vi "SetTriggerDelay.vi"(8 "error in (no error)":errorcluster, 10 "Arg":string, 11 "ThorLabsCsCamera in":refnum<class "ThorLabsCsCamera.lvclass">) -> (0 "error out":errorcluster, 2 "setValue out":dbl, 3 "ThorLabsCsCamera out":refnum<class "ThorLabsCsCamera.lvclass">)   [LabVIEW 2020, in "ThorLabsCsCamera.lvclass"]
uses:
  ThorLabsCsCamera.lvclass
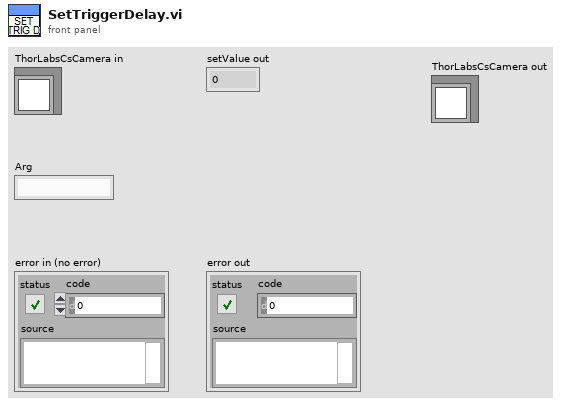
[diagram p1: front panel]
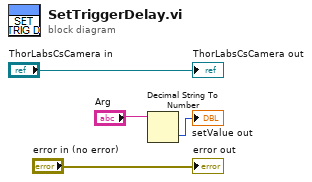
[diagram p0: block diagram]
diagram:
  n1 = Decimal String To Number(string="Arg") -> (number=→"setValue out":i32)  [unwired: 2 in, 1 out]
  "error out" <- "error in (no error)"
  "ThorLabsCsCamera out" <- "ThorLabsCsCamera in"
